vi "Cursor  - Find Position.vi"() -> (1 "Cursor Position":i32[](array[numeric]))   [LabVIEW 2013]
uses:
  USER32.DLL
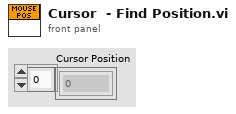
[diagram p1: front panel]
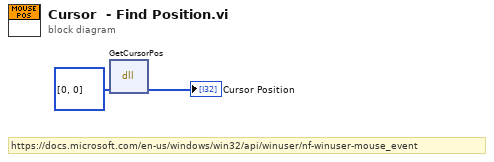
[diagram p0: block diagram]
diagram:
  # "https://docs.microsoft.com/en-us/windows/win32/api/winuser/nf-winuser-mouse_event"
  n1 = dll-call lib="USER32.DLL" fn="GetCursorPos" label="Read Cursor"("Position"=i32[] [0, 0]) -> ("Position"=→"Cursor Position":i32[])  [unwired: 4 in, 2 out]
